vi "FTW-System-CommandLineExecute.vi"(0 "Command":string, 5 "stdin":string, 7 "Working Directory":path, 11 "error in":errorcluster) -> (4 "stdout":string, 15 "error out":errorcluster)   [LabVIEW 2015]
uses:
  lib/ftw32.dll
panel:
  out "Terminating Signal":i64
  out "Return Code":i64
  # "Inputs"
  # "Outputs"
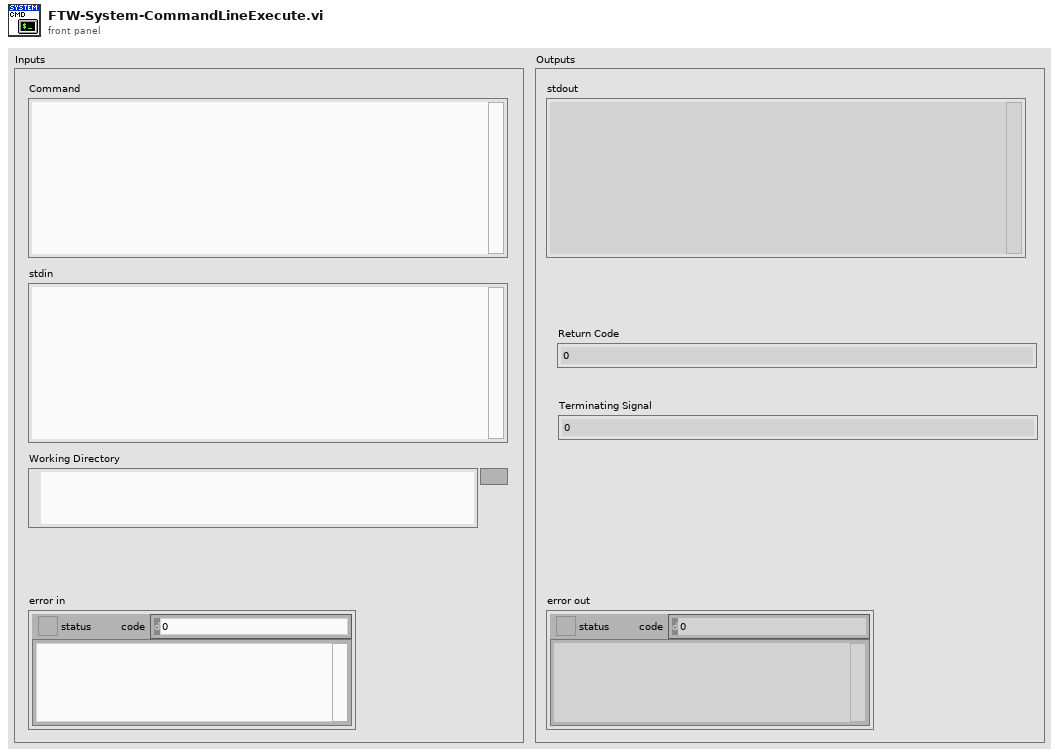
[diagram p1: front panel]
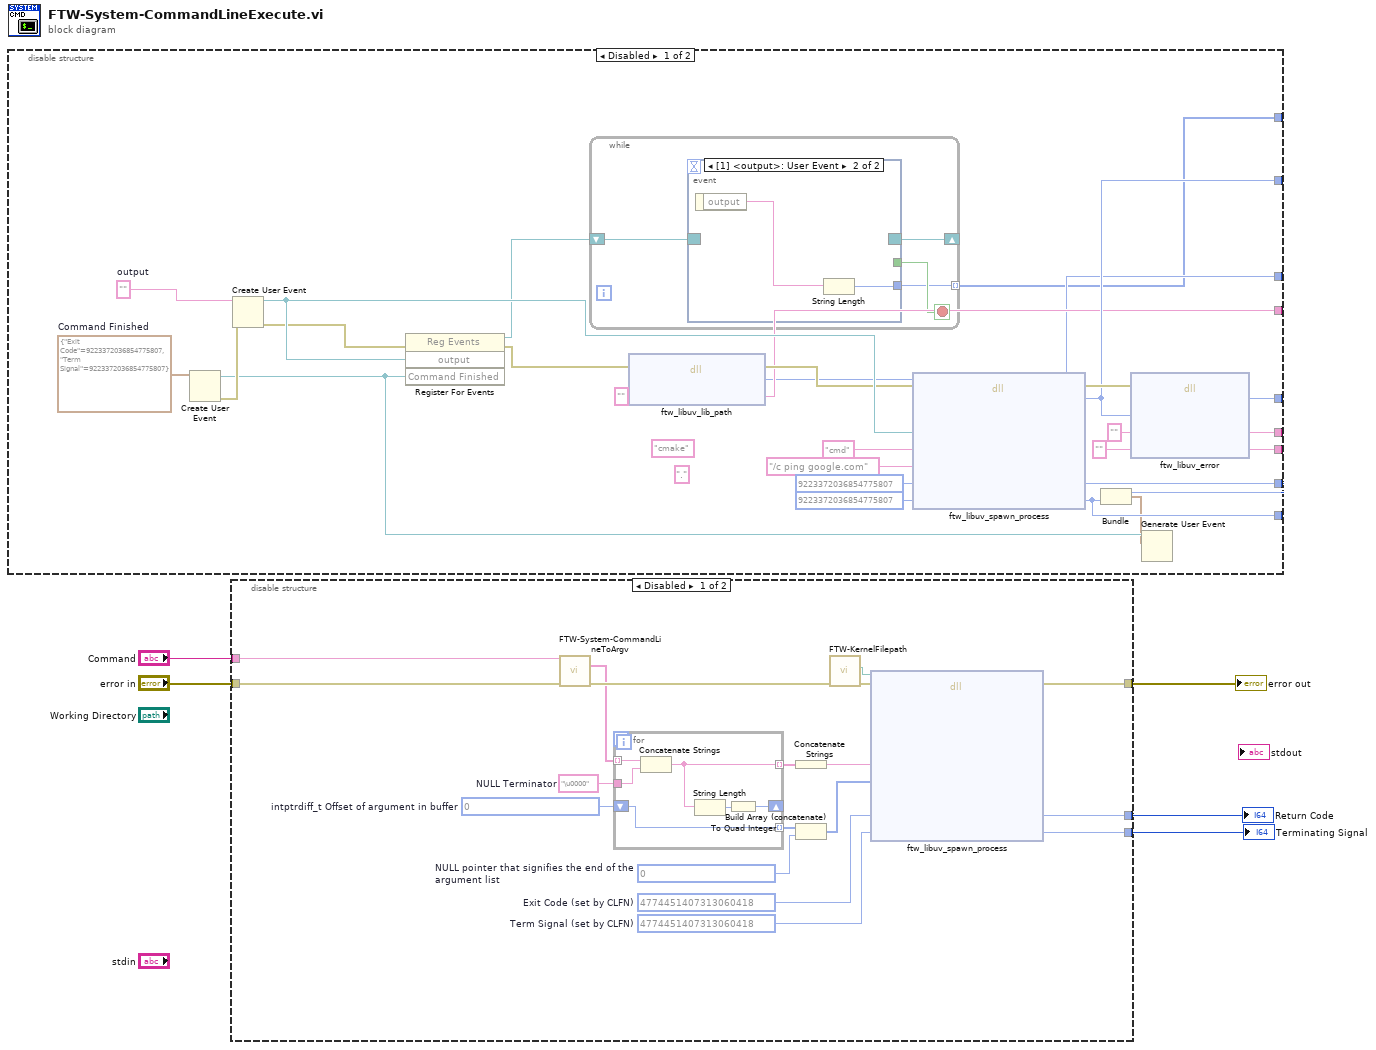
[diagram p0: block diagram]
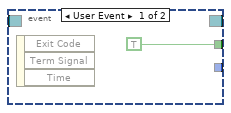
[diagram p2: hidden frame]
diagram:
  n1 = disable-structure shown="Disabled" {
    disable-tunnel: [w30 _] -> _
    disable-tunnel: [w29 _] -> _
    disable-tunnel: [w26 _] -> _
    disable-tunnel: [w25 _] -> _
    disable-tunnel: [w18 _] -> _
    disable-tunnel: [w17 _] -> _
    disable-tunnel: [w16 _] -> _
    disable-tunnel: [w9 _] -> _
    disable-tunnel: [w8 _] -> _
    frame Disabled {
      w6 = ""  # output
      w11 = cluster{"Exit Code":i64, "Term Signal":i64} {"Exit Code"=9223372036854775807, "Term Signal"=9223372036854775807}  # Command Finished
      (unwired) "." ("Arguments")
      (unwired) "cmake" ("Address")
      n2 = Create User Event(user event datatype=w11) -> (user event=w10:refnum<user-event>, error out=w12:errorcluster)  [unwired: 1 in]
      n3 = Create User Event(user event datatype=w6, error in=w12) -> (user event=w23:refnum<user-event>, error out=w13:errorcluster)
      n4 = register-events(error in=w13, w23, w10) -> (reference out=w22:refnum<event-registration>, error out=w21:errorcluster)  [unwired: 1 in]
      n5 = while {
        shift-right: [w34] -> _
        shift-left: w22 -> [w36]
        tunnel: [w33] -> w16 mode=indexing
        stop <- w35 stop-if-true
        n6 = event shown="[1] <output>: User Event" {
          selector: w36 -> [_ _]
          dyn-events: [_ _] -> w34
          timeout: _ -> [_ _]
          tunnel: [TRUE _] -> w35
          tunnel: [_ w38] -> w33
          event User Event {
            n7 = event-data() -> ()  [unwired: 1 in, 3 out]
          }
          event User Event {
            n8 = event-data() -> ("output"=w39:string)  [unwired: 1 in]
            n9 = String Length(string=w39) -> (length=w38:i32)
          }
        }
      }
      n10 = dll-call lib="C:/Users/Jack/repo/featherweight/lib/ftw32.dll" fn="ftw_libuv_lib_path"(error in=w21, "Library Path"="") -> (error out=w20:errorcluster, "Return Value"=w17:i64, "Library Path"=w18:string)  [unwired: 2 in, 1 out]
      n11 = dll-call lib="C:/Users/Jack/repo/featherweight/lib/ftw32.dll" fn="ftw_libuv_spawn_process"(error in=w20, "Output"=w23, "Command"="cmd" ("Address"), "Arguments"="/c ping google.com", "Exit Code"=i64 9223372036854775807, "Term Signal"=i64 9223372036854775807) -> (error out=w31:errorcluster, "Return Value"=w29:i64, "Exit Code"=w9:i64, "Term Signal"=w8:i64)  [unwired: 7 in, 1 out]
      n12 = Bundle("Exit Code"=w9, "Term Signal"=w8) -> (w7:cluster{"Exit Code":i64, "Term Signal":i64})  [unwired: 1 in]
      n13 = dll-call lib="C:/Users/Jack/repo/featherweight/lib/ftw32.dll" fn="ftw_libuv_error"(error in=w31, "Error Code"=w29, "Error Name"="", "Error Description"="") -> ("Return Value"=w30:i64, "Error Name"=w26:string, "Error Description"=w25:string)  [unwired: 3 in, 2 out]
      n14 = Generate User Event(user event=w10, event data cluster=w7) -> ()  [unwired: 2 in, 2 out]
    }
    frame Enabled {
    }
  }
  n15 = disable-structure shown="Disabled" {
    disable-tunnel: "Command" -> [w57 _]
    disable-tunnel: "error in" -> [w53 _]
    disable-tunnel: [w43 _] -> w3
    disable-tunnel: [w42 _] -> w2
    disable-tunnel: [w41 _] -> w1
    frame Disabled {
      w44 = i64 4774451407313060418  # Term Signal (set by CLFN)
      w45 = i64 4774451407313060418  # Exit Code (set by CLFN)
      w47 = i64 0  # NULL pointer that signifies the end of the argument list
      w49 = i64 0  # intptrdiff_t Offset of argument in buffer
      w52 = "\u0000"  # NULL Terminator
      n16 = call "FTW-System-CommandLineToArgv.vi"("Command"=w57, "error in"=w53) -> ("**argv"=w40:string[], "error out"=w55:errorcluster)  [unwired: 12 in]
      n17 = for {
        tunnel: w40 -> [w62] mode=indexing
        tunnel: w52 -> [w63]
        tunnel: [w61] -> w50 mode=indexing
        shift-right: [w59] -> _
        shift-left: w49 -> [w58]
        tunnel: [w58] -> w48 mode=indexing
        n18 = Concatenate Strings(w62, w63) -> (w61:string)
        n19 = String Length(string=w61) -> (length=w60:i32)
        n20 = To Quad Integer(1:w60) -> (0:w59:i64)
      }
      n21 = Concatenate Strings(w50) -> (w51:string)
      n22 = Build Array (concatenate)(w48, w47) -> (w46:i64[])
      n23 = call "FTW-KernelFilepath.vi"("error in"=w55) -> ("error out"=w56:errorcluster, "Library Filepath"=w54:path)  [unwired: 8 in, 1 out]
      n24 = dll-call lib="?" fn="ftw_libuv_spawn_process"(path in=w54, error in=w56, "NULL-delimited Arguments"=w51, "Argument Offsets"=w46, "Exit Code"=w45, "Term Signal"=w44) -> (error out=w41:errorcluster, "Exit Code"=w43:i64, "Term Signal"=w42:i64)  [unwired: 12 in, 1 out]
    }
    frame Enabled {
    }
  }
  "error out" <- w1
  "Return Code" <- w3
  "Terminating Signal" <- w2
